vi "HJ212-2017.vi"(8 "error in (no error)":errorcluster caption="错误输入（无错误）", 11 "数据段":T1) -> (0 "error out":errorcluster caption="错误输出", 2 "通讯包字符串":string, 3 "通讯包":T2={"包头（2）"="##", "数据段长度（4）"="", "数据段"="", "CRC校验"="", "包尾"=""})   [LabVIEW 2016]
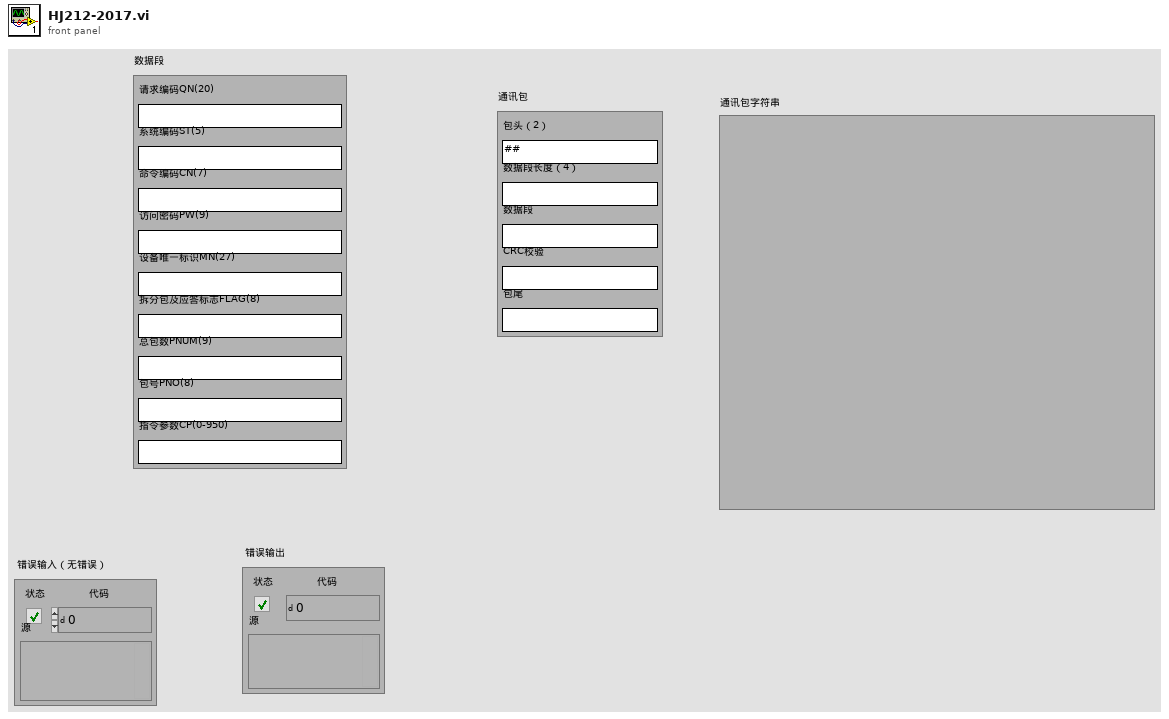
[diagram p1: front panel]
types:
  T1 = cluster{"请求编码QN(20)":string, "系统编码ST(5)":string, "命令编码CN(7)":string, "访问密码PW(9)":string, "设备唯一标识MN(27)":string, "拆分包及应答标志FLAG(8)":string, "总包数PNUM(9)":string, "包号PNO(8)":string, "指令参数CP(0-950)":string}
  T2 = cluster{"包头（2）":string, "数据段长度（4）":string, "数据段":string, "CRC校验":string, "包尾":string}
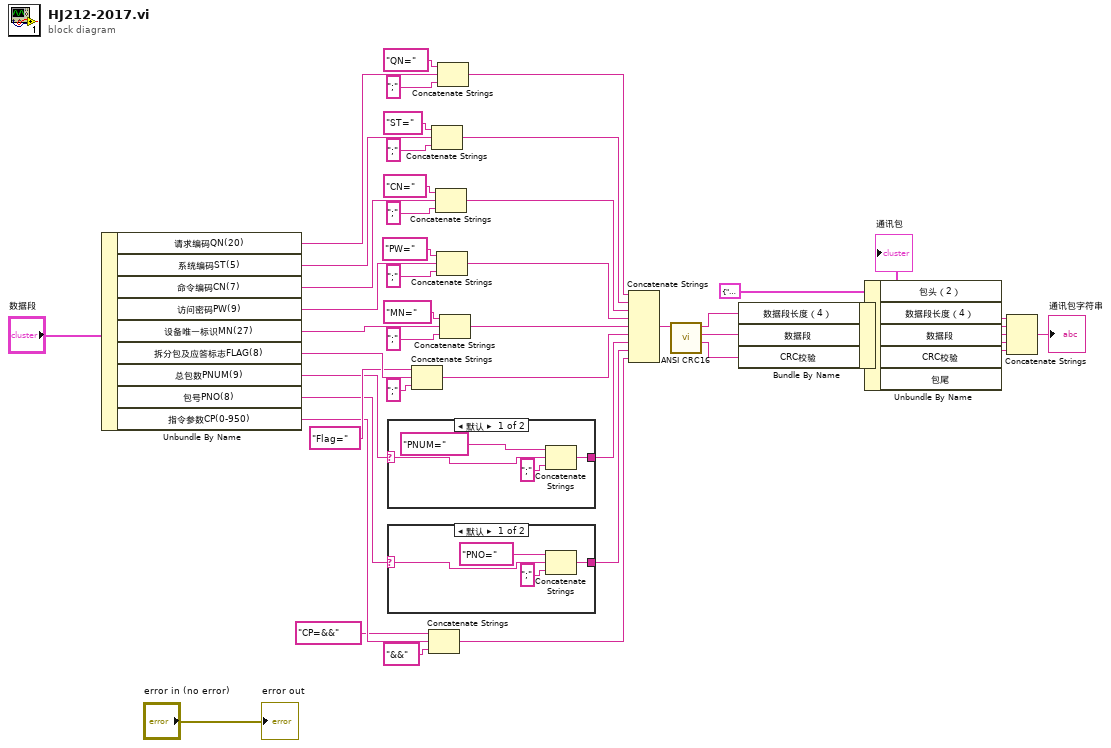
[diagram p0: block diagram]
diagram:
  n1 = Unbundle By Name("数据段") -> ("请求编码QN(20)"=w45:string, "系统编码ST(5)"=w41:string, "命令编码CN(7)"=w39:string, "访问密码PW(9)"=w36:string, "设备唯一标识MN(27)"=w33:string, "拆分包及应答标志FLAG(8)"=w25:string, "总包数PNUM(9)"=w21:string, "包号PNO(8)"=w19:string, "指令参数CP(0-950)"=w17:string)
  n2 = case shown="默认" w21 {
    selector: w21 -> [w49 w51]
    tunnel: [w47 w51] -> w20
    frame Default {
      n3 = Concatenate Strings("PNUM=" ("字符串"), w49, ";" ("字符串")) -> (w47:string)
    }
    frame "" {
    }
  }
  n4 = case shown="默认" w19 {
    selector: w19 -> [w54 w56]
    tunnel: [w52 w56] -> w18
    frame Default {
      n5 = Concatenate Strings("PNO=" ("字符串"), w54, ";" ("字符串")) -> (w52:string)
    }
    frame "" {
    }
  }
  n6 = Concatenate Strings("Flag=" ("字符串"), w25, ";" ("字符串")) -> (w22:string)
  n7 = Concatenate Strings("CP=&&" ("字符串"), w17, "&&" ("字符串")) -> (w14:string)
  n8 = Concatenate Strings("ST=" ("字符串"), w41, ";" ("字符串")) -> (w30:string)
  n9 = Concatenate Strings("CN=" ("字符串"), w39, ";" ("字符串")) -> (w29:string)
  n10 = Concatenate Strings("PW=" ("字符串"), w36, ";" ("字符串")) -> (w28:string)
  n11 = Concatenate Strings("QN=" ("字符串"), w45, ";" ("字符串")) -> (w44:string)
  n12 = Concatenate Strings("MN=" ("字符串"), w33, ";" ("字符串")) -> (w27:string)
  n13 = Concatenate Strings(w44, w30, w29, w28, w27, w22, w20, w18, w14) -> (w13:string)
  n14 = call "ANSI CRC16.vi"("puchMsg"=w13) -> ("CRC校验"=w1:string, "数据段"=w2:string, "数据段长度"=w3:string)  [unwired: 8 in]
  n15 = Bundle By Name(cluster=T2 {"包头（2）"="##", "数据段长度（4）"="", "数据段"="", "CRC校验"="", "包尾"="\r\n"} ("通讯包"), "数据段长度（4）"=w3, "数据段"=w2, "CRC校验"=w1) -> (w10:T2)
  "通讯包" <- w10
  n16 = Unbundle By Name(w10) -> ("包头（2）"=w9:string, "数据段长度（4）"=w8:string, "数据段"=w7:string, "CRC校验"=w6:string, "包尾"=w5:string)
  n17 = Concatenate Strings(w9, w8, w7, w6, w5) -> (→"通讯包字符串":string)
  "error out" <- "error in (no error)"
